vi "Write Start Index.vi"(8 "error in (no error)":errorcluster, 10 "Start Index":i32, 11 "Set Output Values Msg in":refnum<class "Set Output Values Msg.lvclass">) -> (0 "error out":errorcluster, 3 "Set Output Values Msg out":refnum<class "Set Output Values Msg.lvclass">)   [LabVIEW 2020, in "BNT_ULx.lvlib" / "Set Output Values Msg.lvclass"]
uses:
  Set Output Values Msg.lvclass
  Set Output Values Msg.lvclass/Set Output Values Msg.ctl
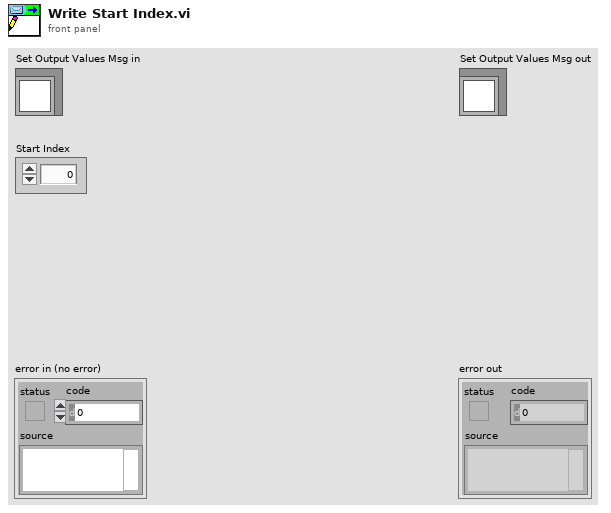
[diagram p1: front panel]
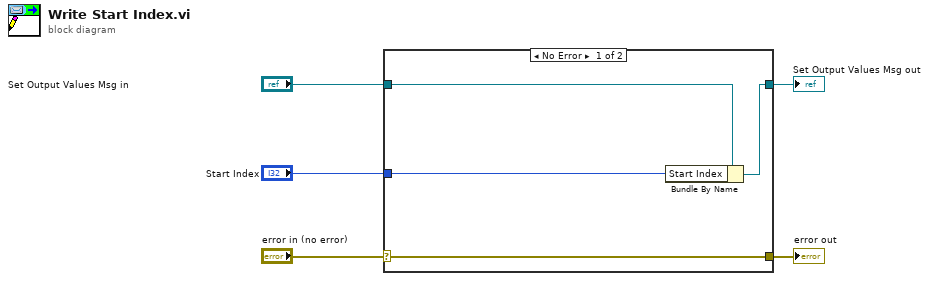
[diagram p0: block diagram]
diagram:
  n1 = case shown="No Error" "error in (no error)" {
    selector: "error in (no error)" -> [w9 w10]
    tunnel: [w9 w10] -> w4
    tunnel: [w7 w11] -> w2
    tunnel: "Set Output Values Msg in" -> [w8 w11]
    tunnel: "Start Index" -> [w6 _]
    frame No Error {
      n2 = Bundle By Name(cluster=w8, "Start Index"=w6) -> (w7:refnum<class "Set Output Values Msg.lvclass">)
    }
    frame Error {
    }
  }
  "error out" <- w4
  "Set Output Values Msg out" <- w2
